vi "Exponential Test.vi"() -> ()   [LabVIEW 2014]
uses:
  <vilib>/Math Plots/3D Math Plots/3D Scatter/3D Scatter XCtrl/3D Scatter.xctl
  <vilib>/Math Plots/3D Math Plots/3D Scatter/3D Scatter Datatype/Public/Plot Helper (Vector).vi
  <vilib>/Analysis/1siggen.llb/Ramp Pattern by Delta.vi
  Math Utilities.lvlib
  <vilib>/Analysis/NI_AALBase.lvlib
  <vilib>/measure/NI_MABase.lvlib
  <vilib>/Math Plots/3D Math Plots/3D Scatter/3D Scatter Datatype/3D Scatter Datatype.lvclass
panel:
  in  "meth":enum8{"DFT-1", "DFT-5", "LRS"}(ring)=enum."LRS" caption="Exponential Fit Method"
  out "etau'":cluster{dbl[], dbl[]}[](graph)=[{[0.0, 0.05, 0.1, 0.15, 0.2, 0.25, 0.3, 0.35, 0.4, 0.45, 0.5, 0.55, 0.6, 0.65, 0.7, 0.75, 0.8, 0.85, 0.9, 0.95, 1.0, 1.05, 1.1, 1.15, 1.2, 1.25, 1.3, 1.35, 1.4, 1.45, 1.5, 1.55, 1.6, 1.65, 1.7, 1.75, 1.8, 1.85, 1.9, 1.95, 2.0, 2.05, 2.1, 2.15, 2.2, 2.25, 2.3, 2.35, 2.4, 2.45, 2.5, 2.55, 2.6, 2.65, 2.7, 2.75, 2.8, 2.85, 2.9, 2.95, 3.0, 3.05, 3.1, 3.15, 3.2, 3.25, 3.3, 3.35, 3.4, 3.45, 3.5, 3.55, 3.6, 3.65, 3.7, 3.75, 3.8, 3.85, 3.9, 3.95, 4.0, 4.05, 4.1, 4.15, 4.2, 4.25, 4.3, 4.35, 4.4, 4.45, 4.5, 4.55, 4.6, 4.65, 4.7, 4.75, 4.8, 4.85, 4.9, 4.95], [0.960541444934628, 1.0300287046137588, 0.8896412059372913, 0.8809320306793802, 0.7883247330312061, 0.8176833763391205, 0.6447128922258879, 0.6273332809368509, 0.6605682518837364, 0.6670014264280115, 0.583805564940926, 0.675732358744051, 0.4639846933111526, 0.6202542521121932, 0.5597277145279371, 0.5135564243561868, 0.5062733727780937, 0.3613578160271843, 0.4475233678516537, 0.3793968608808492, 0.43724877411342006, 0.3597384315625127, 0.2373620816547545, 0.22453592933762084, 0.29842459974751334, 0.3050071640074105, 0.2359236866011837, 0.24302284161365773, 0.23920428907537397, 0.2700720254736181, 0.1918881215092269, 0.2316375620963971, 0.2698374059004593, 0.10938565371609907, 0.18228368619733432, 0.1995904055680095, 0.10262683454287629, 0.12951323626014882, 0.1883316121198414, 0.051005880662942066, 0.1882658145929273, 0.2253474344702741, 0.1072676376138868, 0.05420331503554107, 0.07073686122149538, 0.19072834912888081, 0.06489404614590896, 0.02340665923857653, 0.080727031502262, 0.053160478621205834, 0.1150566849039812, 0.08647339206694683, 0.17225004999139676, 0.14385515421965545, 0.09476811084635094, 0.08535850566392958, 0.042453337460426295, -0.005111835078437502, 0.1266720101202937, 0.08798857698089546, 0.06448330591172151, 0.012535109492323698, -0.02180050629331399, 0.13921091410606592, -0.00448119475112807, 0.025953771409014427, 0.09196924940378937, 0.1251848736523793, 0.09872337746996236, -0.02796928416987523, -0.0439093646999277, 0.07577564143222511, -0.03469012345164275, 0.1000290582787502, 0.07570130581455305, 0.10981843839037647, 0.030883562880611268, 0.05482327411195698, -0.016277970417741722, 0.0739773731669493, 0.11823230258380474, 0.022378034520468177, 0.015118202748243353, 0.06436576688809863, 0.034369714129696256, -0.07590989562072355, 0.11223730777048424, -0.05352288298618646, 0.059251144916092124, -0.054463595365239675, 0.10903521158421503, 0.07349724843361212, -0.04763649889666532, 0.05840026342982382, -0.06312941047179772, -0.04841695002411584, 0.0871009289199655, -0.08241366972549377, 0.06657825659960447, 0.01870496404000565]}, {[0.0, 0.1, 0.2, 0.3, 0.4, 0.5, 0.6, 0.7, 0.8, 0.9, 1.0, 1.1, 1.2, 1.3, 1.4, 1.5, 1.6, 1.7, 1.8, 1.9, 2.0, 2.1, 2.2, 2.3, 2.4, 2.5, 2.6, 2.7, 2.8, 2.9, 3.0, 3.1, 3.2, 3.3, 3.4, 3.5, 3.6, 3.7, 3.8, 3.9, 4.0, 4.1, 4.2, 4.3, 4.4, 4.5, 4.6, 4.7, 4.8, 4.9], [1.0489118049155677, 0.9828657414468108, 0.7287092685494896, 0.7402604459878791, 0.5870346294794287, 0.586721816909444, 0.45440624030548527, 0.5237279303930864, 0.3972561140761981, 0.33254829917367884, 0.34818621735970484, 0.3989198005547301, 0.34947614865970883, 0.20883760536624074, 0.20965525245589398, 0.26857776347019313, 0.23122560558625996, 0.23874984457269088, 0.15561255360224382, 0.1418318343504817, 0.11626272362059906, 0.16392580193843515, 0.033834333279495796, 0.0778706880250746, -0.007929789367372514, 0.005419938340864641, 0.04836411782582296, 0.12887685022889384, 0.15987281329989583, 0.002826123372845442, 0.044361005460079386, 0.01107762227846102, 0.027130325332161268, -0.0329011607483985, -0.00976715691082395, -0.01851382955827155, -0.02912386416561294, 0.05216385233514075, -0.01890067181650635, -0.06324219670124576, -0.06851294508129749, -0.002777132357630538, -0.014512361417010615, 0.08683899542703284, 0.08258002031887463, -0.024344103284262092, 0.0437718075673618, -0.06155030056137617, 0.06644365751447188, 0.05045892575985402]}, {[0.0, 0.2, 0.4, 0.6, 0.8, 1.0, 1.2, 1.4, 1.6, 1.8, 2.0, 2.2, 2.4, 2.6, 2.8, 3.0, 3.2, 3.4, 3.6, 3.8, 4.0, 4.2, 4.4, 4.6, 4.8], [1.0166445888668472, 0.8965127205564365, 0.6746646020918559, 0.5979355379266843, 0.4854152133224972, 0.3872720439703156, 0.3657660253817956, 0.30351089738058307, 0.2198216708301479, 0.20705366479755255, 0.06903085210606028, 0.16530276730729707, 0.15939586940300982, 0.083518667159258, 0.0640925481270926, 0.06369433525293566, 0.04352509905837727, 0.036281546977637566, 0.043303657543107665, 0.08611682194308087, 0.029590496545093097, -0.01733169050921223, -0.024397551503856203, -0.05234666017391198, -0.03711380387257694]}, {[0.0, 0.5, 1.0, 1.5, 2.0, 2.5, 3.0, 3.5, 4.0, 4.5], [1.0623034361710997, 0.5317673867138099, 0.42771698929286195, 0.17661929472640508, 0.05033997654512429, 0.03973823954012479, 0.09664850852882598, 0.07924682307796599, 0.11213514888422532, 0.10083456799625037]}, {[0.0, 1.0, 2.0, 3.0, 4.0], [1.097092230716005, 0.32607780199041114, 0.13609726715261378, 0.0013463089040823967, 0.0574822313090591]}]
  out "tau'":cluster{dbl[], dbl[]}[](graph)=[{[0.0, 0.05, 0.1, 0.15, 0.2, 0.25, 0.3, 0.35, 0.4, 0.45, 0.5, 0.55, 0.6, 0.65, 0.7, 0.75, 0.8, 0.85, 0.9, 0.95, 1.0, 1.05, 1.1, 1.15, 1.2, 1.25, 1.3, 1.35, 1.4, 1.45, 1.5, 1.55, 1.6, 1.65, 1.7, 1.75, 1.8, 1.85, 1.9, 1.95, 2.0, 2.05, 2.1, 2.15, 2.2, 2.25, 2.3, 2.35, 2.4, 2.45, 2.5, 2.55, 2.6, 2.65, 2.7, 2.75, 2.8, 2.85, 2.9, 2.95, 3.0, 3.05, 3.1, 3.15, 3.2, 3.25, 3.3, 3.35, 3.4, 3.45, 3.5, 3.55, 3.6, 3.65, 3.7, 3.75, 3.8, 3.85, 3.9, 3.95, 4.0, 4.05, 4.1, 4.15, 4.2, 4.25, 4.3, 4.35, 4.4, 4.45, 4.5, 4.55, 4.6, 4.65, 4.7, 4.75, 4.8, 4.85, 4.9, 4.95], [0.960541444934628, 1.0300287046137588, 0.8896412059372913, 0.8809320306793802, 0.7883247330312061, 0.8176833763391205, 0.6447128922258879, 0.6273332809368509, 0.6605682518837364, 0.6670014264280115, 0.583805564940926, 0.675732358744051, 0.4639846933111526, 0.6202542521121932, 0.5597277145279371, 0.5135564243561868, 0.5062733727780937, 0.3613578160271843, 0.4475233678516537, 0.3793968608808492, 0.43724877411342006, 0.3597384315625127, 0.2373620816547545, 0.22453592933762084, 0.29842459974751334, 0.3050071640074105, 0.2359236866011837, 0.24302284161365773, 0.23920428907537397, 0.2700720254736181, 0.1918881215092269, 0.2316375620963971, 0.2698374059004593, 0.10938565371609907, 0.18228368619733432, 0.1995904055680095, 0.10262683454287629, 0.12951323626014882, 0.1883316121198414, 0.051005880662942066, 0.1882658145929273, 0.2253474344702741, 0.1072676376138868, 0.05420331503554107, 0.07073686122149538, 0.19072834912888081, 0.06489404614590896, 0.02340665923857653, 0.080727031502262, 0.053160478621205834, 0.1150566849039812, 0.08647339206694683, 0.17225004999139676, 0.14385515421965545, 0.09476811084635094, 0.08535850566392958, 0.042453337460426295, -0.005111835078437502, 0.1266720101202937, 0.08798857698089546, 0.06448330591172151, 0.012535109492323698, -0.02180050629331399, 0.13921091410606592, -0.00448119475112807, 0.025953771409014427, 0.09196924940378937, 0.1251848736523793, 0.09872337746996236, -0.02796928416987523, -0.0439093646999277, 0.07577564143222511, -0.03469012345164275, 0.1000290582787502, 0.07570130581455305, 0.10981843839037647, 0.030883562880611268, 0.05482327411195698, -0.016277970417741722, 0.0739773731669493, 0.11823230258380474, 0.022378034520468177, 0.015118202748243353, 0.06436576688809863, 0.034369714129696256, -0.07590989562072355, 0.11223730777048424, -0.05352288298618646, 0.059251144916092124, -0.054463595365239675, 0.10903521158421503, 0.07349724843361212, -0.04763649889666532, 0.05840026342982382, -0.06312941047179772, -0.04841695002411584, 0.0871009289199655, -0.08241366972549377, 0.06657825659960447, 0.01870496404000565]}, {[0.0, 0.1, 0.2, 0.3, 0.4, 0.5, 0.6, 0.7, 0.8, 0.9, 1.0, 1.1, 1.2, 1.3, 1.4, 1.5, 1.6, 1.7, 1.8, 1.9, 2.0, 2.1, 2.2, 2.3, 2.4, 2.5, 2.6, 2.7, 2.8, 2.9, 3.0, 3.1, 3.2, 3.3, 3.4, 3.5, 3.6, 3.7, 3.8, 3.9, 4.0, 4.1, 4.2, 4.3, 4.4, 4.5, 4.6, 4.7, 4.8, 4.9], [1.0489118049155677, 0.9828657414468108, 0.7287092685494896, 0.7402604459878791, 0.5870346294794287, 0.586721816909444, 0.45440624030548527, 0.5237279303930864, 0.3972561140761981, 0.33254829917367884, 0.34818621735970484, 0.3989198005547301, 0.34947614865970883, 0.20883760536624074, 0.20965525245589398, 0.26857776347019313, 0.23122560558625996, 0.23874984457269088, 0.15561255360224382, 0.1418318343504817, 0.11626272362059906, 0.16392580193843515, 0.033834333279495796, 0.0778706880250746, -0.007929789367372514, 0.005419938340864641, 0.04836411782582296, 0.12887685022889384, 0.15987281329989583, 0.002826123372845442, 0.044361005460079386, 0.01107762227846102, 0.027130325332161268, -0.0329011607483985, -0.00976715691082395, -0.01851382955827155, -0.02912386416561294, 0.05216385233514075, -0.01890067181650635, -0.06324219670124576, -0.06851294508129749, -0.002777132357630538, -0.014512361417010615, 0.08683899542703284, 0.08258002031887463, -0.024344103284262092, 0.0437718075673618, -0.06155030056137617, 0.06644365751447188, 0.05045892575985402]}, {[0.0, 0.2, 0.4, 0.6, 0.8, 1.0, 1.2, 1.4, 1.6, 1.8, 2.0, 2.2, 2.4, 2.6, 2.8, 3.0, 3.2, 3.4, 3.6, 3.8, 4.0, 4.2, 4.4, 4.6, 4.8], [1.0166445888668472, 0.8965127205564365, 0.6746646020918559, 0.5979355379266843, 0.4854152133224972, 0.3872720439703156, 0.3657660253817956, 0.30351089738058307, 0.2198216708301479, 0.20705366479755255, 0.06903085210606028, 0.16530276730729707, 0.15939586940300982, 0.083518667159258, 0.0640925481270926, 0.06369433525293566, 0.04352509905837727, 0.036281546977637566, 0.043303657543107665, 0.08611682194308087, 0.029590496545093097, -0.01733169050921223, -0.024397551503856203, -0.05234666017391198, -0.03711380387257694]}, {[0.0, 0.5, 1.0, 1.5, 2.0, 2.5, 3.0, 3.5, 4.0, 4.5], [1.0623034361710997, 0.5317673867138099, 0.42771698929286195, 0.17661929472640508, 0.05033997654512429, 0.03973823954012479, 0.09664850852882598, 0.07924682307796599, 0.11213514888422532, 0.10083456799625037]}, {[0.0, 1.0, 2.0, 3.0, 4.0], [1.097092230716005, 0.32607780199041114, 0.13609726715261378, 0.0013463089040823967, 0.0574822313090591]}]
  out "3D Scatter":refnum<class "3D Plot Datatype.lvclass">[](xcontrol)
  out "CalcData":T1(array[cluster])
  in  "taus":dbl[](array[numeric])=[0.5, 1.0, 2.0, 5.0, 10.0, 20.0, 50.0, 100.0, 150.0] caption="taus (us)"
  in  "noise":dbl[](array[numeric])=[0.0, 0.01, 0.05, 0.1, 0.2, 0.3, 0.4, 0.5, 1.0] caption="Noise Levels"
  in  "Ntaus":dbl=5.0 caption="# Taus"
  in  "Nsamp":dbl=4000.0 caption="Number of Samples"
  out "Taus":T2(graph)=[{"Sampling Frequencies (MHz)"=[20.0, 10.0, 5.0, 2.0, 1.0], [0.9656086307823587, 0.9866685202887719, 1.1569644501410312, 0.7662051282812012, 0.8285928880796682]}, {"Sampling Frequencies (MHz)"=[20.0, 10.0, 5.0, 2.0, 1.0], [0.026104009183676023, 0.034896410998791996, 0.03328061139393245, 0.07782595805221088, 0.07635392209771198]}, {"Sampling Frequencies (MHz)"=[20.0, 10.0, 5.0, 2.0, 1.0], [0.9408079235146063, 0.9408079235146063, 0.9408079235146063, 0.9408079235146063, 0.9408079235146063]}]
  out "Exponential":cluster{dbl[], dbl[]}[](graph)=[{[0.0, 0.05, 0.1, 0.15, 0.2, 0.25, 0.3, 0.35, 0.4, 0.45, 0.5, 0.55, 0.6, 0.65, 0.7, 0.75, 0.8, 0.85, 0.9, 0.95, 1.0, 1.05, 1.1, 1.15, 1.2, 1.25, 1.3, 1.35, 1.4, 1.45, 1.5, 1.55, 1.6, 1.65, 1.7, 1.75, 1.8, 1.85, 1.9, 1.95, 2.0, 2.05, 2.1, 2.15, 2.2, 2.25, 2.3, 2.35, 2.4, 2.45, 2.5, 2.55, 2.6, 2.65, 2.7, 2.75, 2.8, 2.85, 2.9, 2.95, 3.0, 3.05, 3.1, 3.15, 3.2, 3.25, 3.3, 3.35, 3.4, 3.45, 3.5, 3.55, 3.6, 3.65, 3.7, 3.75, 3.8, 3.85, 3.9, 3.95, 4.0, 4.05, 4.1, 4.15, 4.2, 4.25, 4.3, 4.35, 4.4, 4.45, 4.5, 4.55, 4.6, 4.65, 4.7, 4.75, 4.8, 4.85, 4.9, 4.95], [0.960541444934628, 1.0300287046137588, 0.8896412059372913, 0.8809320306793802, 0.7883247330312061, 0.8176833763391205, 0.6447128922258879, 0.6273332809368509, 0.6605682518837364, 0.6670014264280115, 0.583805564940926, 0.675732358744051, 0.4639846933111526, 0.6202542521121932, 0.5597277145279371, 0.5135564243561868, 0.5062733727780937, 0.3613578160271843, 0.4475233678516537, 0.3793968608808492, 0.43724877411342006, 0.3597384315625127, 0.2373620816547545, 0.22453592933762084, 0.29842459974751334, 0.3050071640074105, 0.2359236866011837, 0.24302284161365773, 0.23920428907537397, 0.2700720254736181, 0.1918881215092269, 0.2316375620963971, 0.2698374059004593, 0.10938565371609907, 0.18228368619733432, 0.1995904055680095, 0.10262683454287629, 0.12951323626014882, 0.1883316121198414, 0.051005880662942066, 0.1882658145929273, 0.2253474344702741, 0.1072676376138868, 0.05420331503554107, 0.07073686122149538, 0.19072834912888081, 0.06489404614590896, 0.02340665923857653, 0.080727031502262, 0.053160478621205834, 0.1150566849039812, 0.08647339206694683, 0.17225004999139676, 0.14385515421965545, 0.09476811084635094, 0.08535850566392958, 0.042453337460426295, -0.005111835078437502, 0.1266720101202937, 0.08798857698089546, 0.06448330591172151, 0.012535109492323698, -0.02180050629331399, 0.13921091410606592, -0.00448119475112807, 0.025953771409014427, 0.09196924940378937, 0.1251848736523793, 0.09872337746996236, -0.02796928416987523, -0.0439093646999277, 0.07577564143222511, -0.03469012345164275, 0.1000290582787502, 0.07570130581455305, 0.10981843839037647, 0.030883562880611268, 0.05482327411195698, -0.016277970417741722, 0.0739773731669493, 0.11823230258380474, 0.022378034520468177, 0.015118202748243353, 0.06436576688809863, 0.034369714129696256, -0.07590989562072355, 0.11223730777048424, -0.05352288298618646, 0.059251144916092124, -0.054463595365239675, 0.10903521158421503, 0.07349724843361212, -0.04763649889666532, 0.05840026342982382, -0.06312941047179772, -0.04841695002411584, 0.0871009289199655, -0.08241366972549377, 0.06657825659960447, 0.01870496404000565]}, {[0.0, 0.1, 0.2, 0.3, 0.4, 0.5, 0.6, 0.7, 0.8, 0.9, 1.0, 1.1, 1.2, 1.3, 1.4, 1.5, 1.6, 1.7, 1.8, 1.9, 2.0, 2.1, 2.2, 2.3, 2.4, 2.5, 2.6, 2.7, 2.8, 2.9, 3.0, 3.1, 3.2, 3.3, 3.4, 3.5, 3.6, 3.7, 3.8, 3.9, 4.0, 4.1, 4.2, 4.3, 4.4, 4.5, 4.6, 4.7, 4.8, 4.9], [1.0489118049155677, 0.9828657414468108, 0.7287092685494896, 0.7402604459878791, 0.5870346294794287, 0.586721816909444, 0.45440624030548527, 0.5237279303930864, 0.3972561140761981, 0.33254829917367884, 0.34818621735970484, 0.3989198005547301, 0.34947614865970883, 0.20883760536624074, 0.20965525245589398, 0.26857776347019313, 0.23122560558625996, 0.23874984457269088, 0.15561255360224382, 0.1418318343504817, 0.11626272362059906, 0.16392580193843515, 0.033834333279495796, 0.0778706880250746, -0.007929789367372514, 0.005419938340864641, 0.04836411782582296, 0.12887685022889384, 0.15987281329989583, 0.002826123372845442, 0.044361005460079386, 0.01107762227846102, 0.027130325332161268, -0.0329011607483985, -0.00976715691082395, -0.01851382955827155, -0.02912386416561294, 0.05216385233514075, -0.01890067181650635, -0.06324219670124576, -0.06851294508129749, -0.002777132357630538, -0.014512361417010615, 0.08683899542703284, 0.08258002031887463, -0.024344103284262092, 0.0437718075673618, -0.06155030056137617, 0.06644365751447188, 0.05045892575985402]}, {[0.0, 0.2, 0.4, 0.6, 0.8, 1.0, 1.2, 1.4, 1.6, 1.8, 2.0, 2.2, 2.4, 2.6, 2.8, 3.0, 3.2, 3.4, 3.6, 3.8, 4.0, 4.2, 4.4, 4.6, 4.8], [1.0166445888668472, 0.8965127205564365, 0.6746646020918559, 0.5979355379266843, 0.4854152133224972, 0.3872720439703156, 0.3657660253817956, 0.30351089738058307, 0.2198216708301479, 0.20705366479755255, 0.06903085210606028, 0.16530276730729707, 0.15939586940300982, 0.083518667159258, 0.0640925481270926, 0.06369433525293566, 0.04352509905837727, 0.036281546977637566, 0.043303657543107665, 0.08611682194308087, 0.029590496545093097, -0.01733169050921223, -0.024397551503856203, -0.05234666017391198, -0.03711380387257694]}, {[0.0, 0.5, 1.0, 1.5, 2.0, 2.5, 3.0, 3.5, 4.0, 4.5], [1.0623034361710997, 0.5317673867138099, 0.42771698929286195, 0.17661929472640508, 0.05033997654512429, 0.03973823954012479, 0.09664850852882598, 0.07924682307796599, 0.11213514888422532, 0.10083456799625037]}, {[0.0, 1.0, 2.0, 3.0, 4.0], [1.097092230716005, 0.32607780199041114, 0.13609726715261378, 0.0013463089040823967, 0.0574822313090591]}]
  in  "B":dbl
  in  "A":dbl=1.0
  in  "fsamp":dbl[](array[numeric])=[20.0, 15.0, 10.0, 8.0, 6.0, 5.0, 2.5, 1.0] caption="Sampling Frequencies (MHz)"
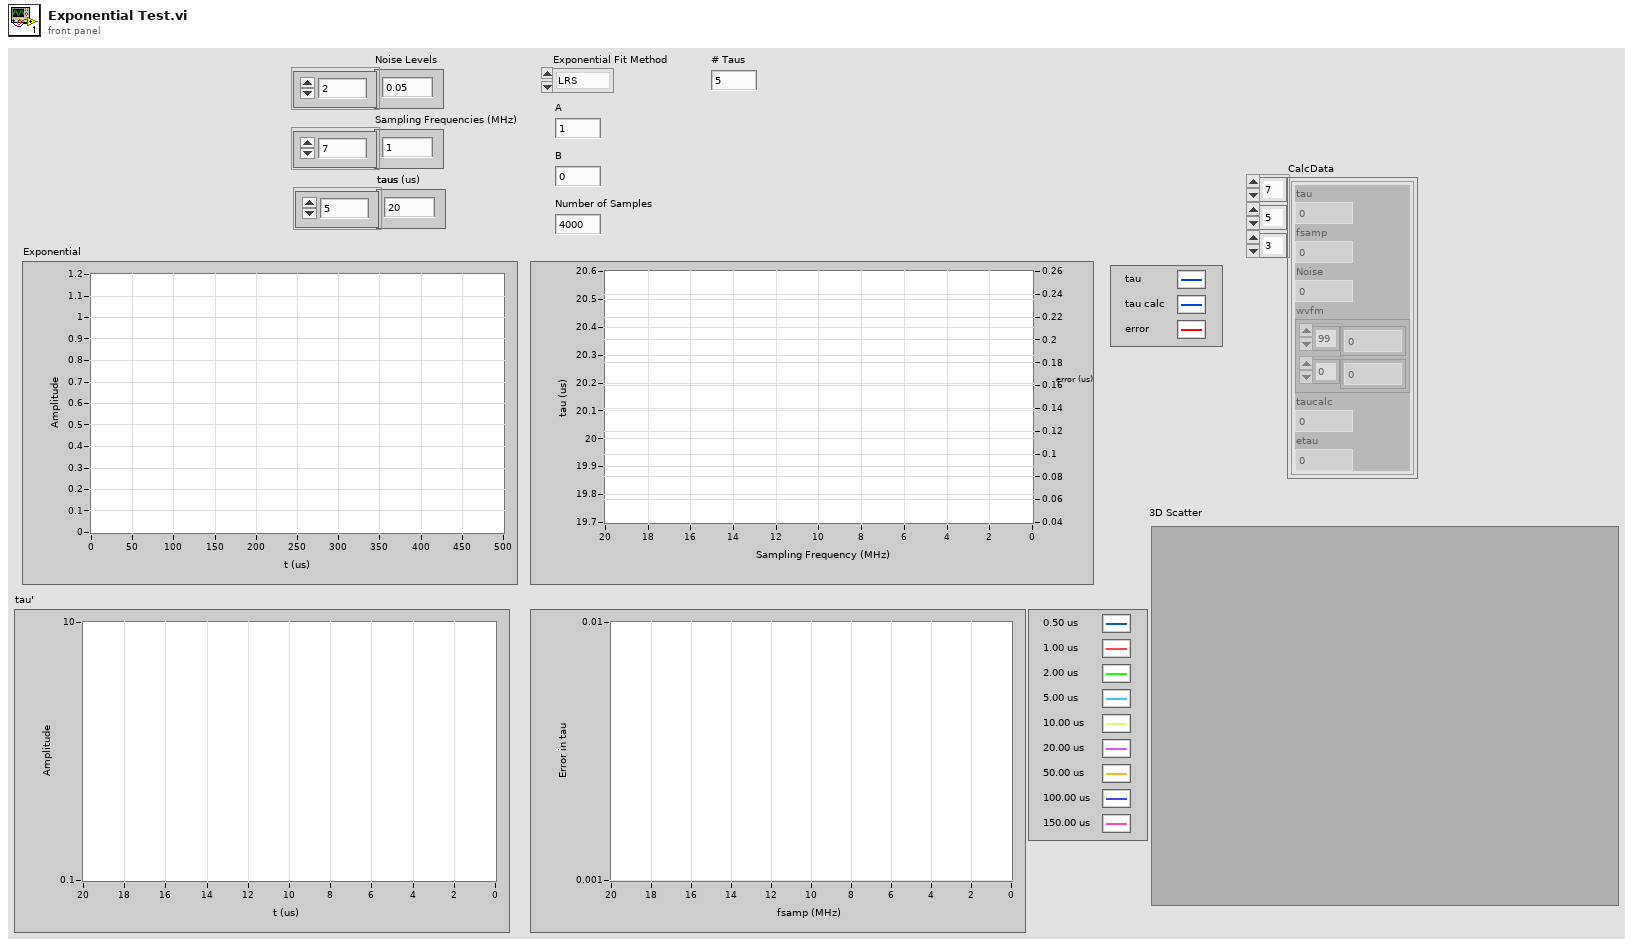
[diagram p1: front panel]
types:
  T1 = cluster{"tau":dbl, "fsamp":dbl, "Noise":dbl, "wvfm":cluster{dbl[], dbl[]}, "taucalc":dbl, "etau":dbl}[][][]
  T2 = cluster{"Sampling Frequencies (MHz)":dbl[], dbl[]}[]
  T3 = cluster{dbl, dbl, "Numeric":dbl, cluster{dbl[], dbl[]}, "tau":dbl, "e_tau":dbl}[][][]
  T4 = cluster{"tau":dbl, "fsamp":dbl, "Noise":dbl, "wvfm":cluster{dbl[], dbl[]}, "taucalc":dbl, "etau":dbl}
  T5 = cluster{"tau":dbl, "fsamp":dbl, "Noise":dbl, "wvfm":cluster{dbl[], dbl[]}, "taucalc":dbl, "etau":dbl}[][]
  T6 = cluster{"tau":dbl, "fsamp":dbl, "Noise":dbl, "wvfm":cluster{dbl[], dbl[]}, "taucalc":dbl, "etau":dbl}[]
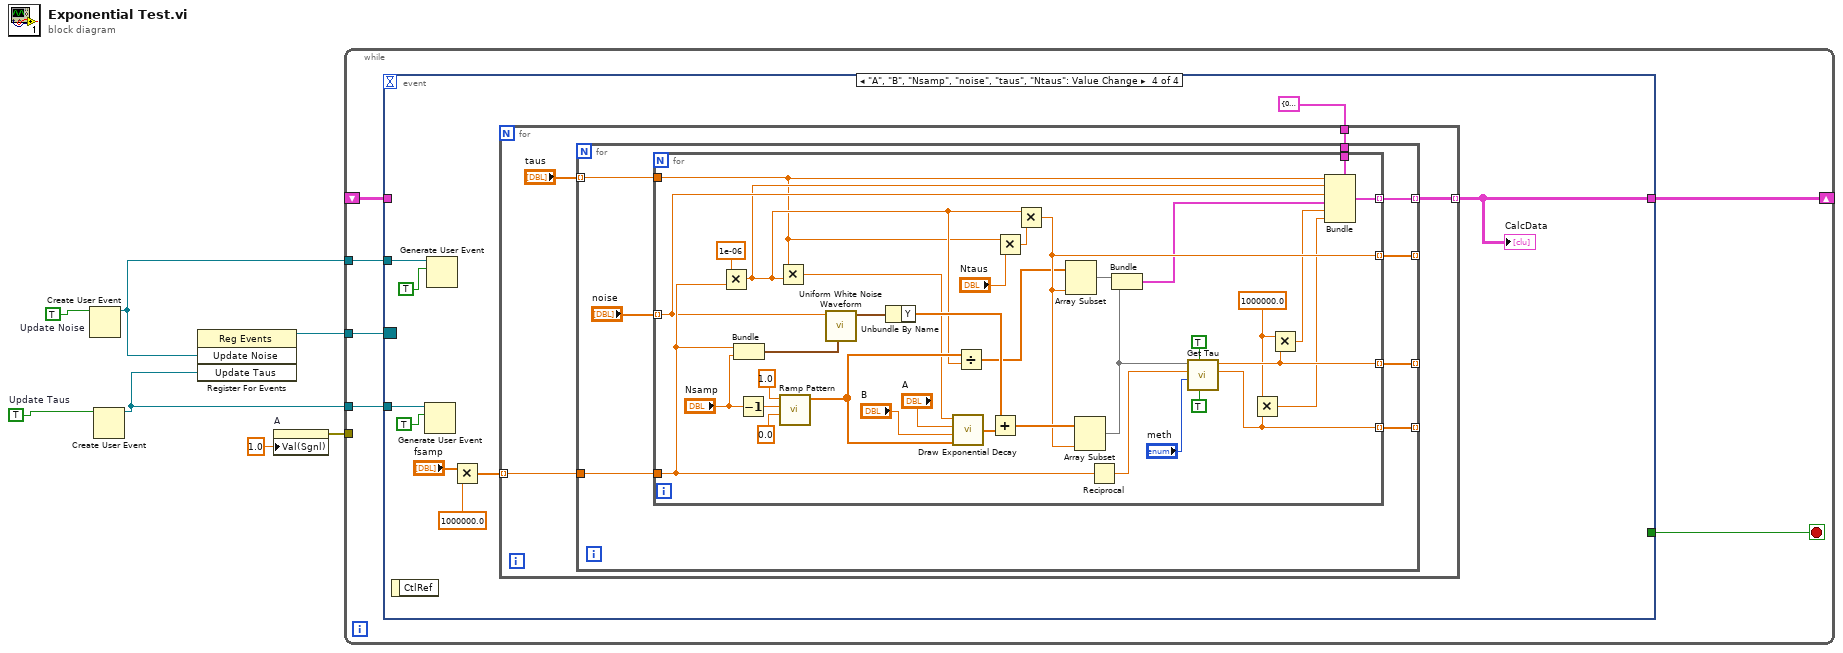
[diagram p0: block diagram]
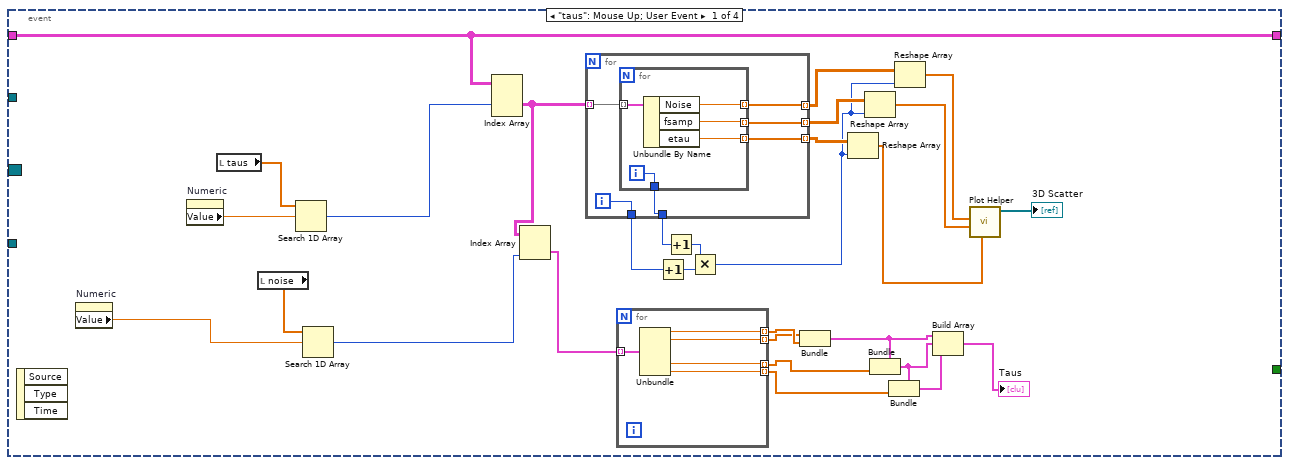
[diagram p2: hidden frame]
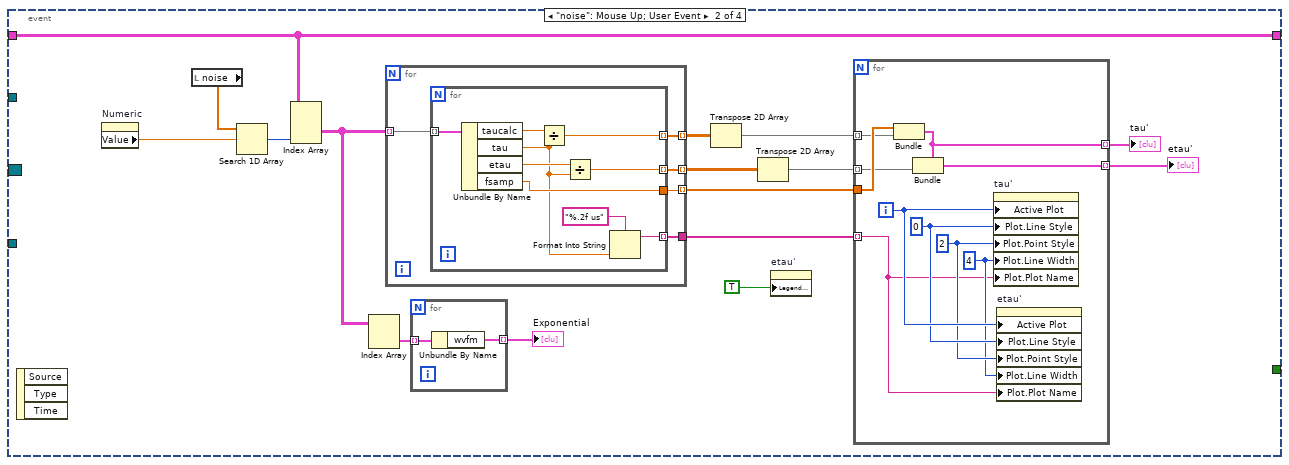
[diagram p3: hidden frame]
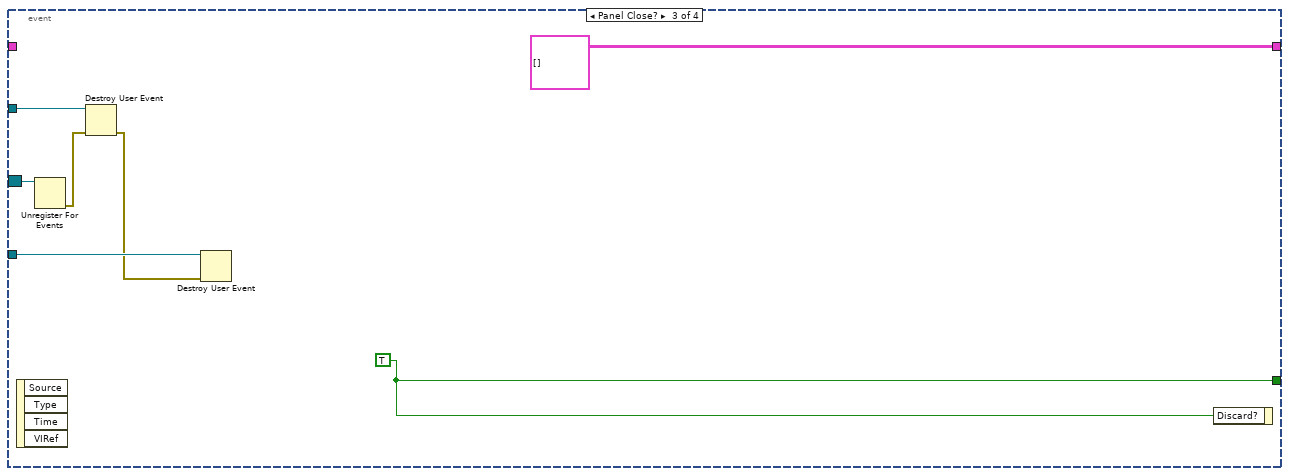
[diagram p4: hidden frame]
diagram:
  w2 = TRUE  # Update Taus
  w5 = TRUE  # Update Noise
  n1 = Create User Event(user event datatype=w5) -> (user event=w3:refnum<user-event>)  [unwired: 1 in, 1 out]
  n2 = Create User Event(user event datatype=w2) -> (user event=w1:refnum<user-event>)  [unwired: 1 in, 1 out]
  n3 = register-events(w3, w1) -> (reference out=w4:refnum<event-registration>)  [unwired: 2 in, 1 out]
  n4 = property on="A" class="DigNum (strict)"("Val(Sgnl)"=1.0 ("Value (Signaling)")) -> (error out=w6:errorcluster)  [unwired: 2 in, 1 out]
  n5 = while {
    shift-right: [w12] -> _
    shift-left: _ -> [w11]
    tunnel: w6 -> [_]
    tunnel: w4 -> [w10]
    tunnel: w3 -> [w9]
    tunnel: w1 -> [w8]
    stop <- w13 stop-if-true
    n6 = event shown="[3] \"A\", \"B\", \"Nsamp\", \"noise\", \"taus\", \"Ntaus\": Value Change" {
      selector: w10 -> [_ _ w103 _]
      dyn-events: _ -> [_ _ _ _]
      timeout: _ -> [_ _ _ _]
      tunnel: [_ _ w107 _] -> w13
      tunnel: [w42 w74 T3 [] w111] -> w12
      tunnel: w11 -> [w42 w74 _ _]
      tunnel: w9 -> [_ _ w104 w113]
      tunnel: w8 -> [_ _ w105 w110]
      event "taus": Mouse Up; User Event {
        n7 = event-data() -> ()  [unwired: 1 in, 3 out]
        n8 = property on="Numeric" class="DigNum (strict)"() -> ("Value"=w26:dbl)  [unwired: 2 in, 2 out]
        n9 = property on="Numeric" class="DigNum (strict)"() -> ("Value"=w28:dbl)  [unwired: 2 in, 2 out]
        n10 = local read "taus"() -> (w29:dbl[])
        n11 = local read "noise"() -> (w25:dbl[])
        n12 = Search 1D Array(1D array=w29, element=w28) -> (index of element=w27:i32)  [unwired: 1 in]
        n13 = Search 1D Array(1D array=w25, element=w26) -> (index of element=w23:i32)  [unwired: 1 in]
        n14 = Index Array(array=w42, index (dim 1)=w27) -> (element=w24:T5)  [unwired: 2 in]
        n15 = Index Array(array=w24, index (col)=w23) -> (element=w22:T6)  [unwired: 1 in]
        n16 = for {
          tunnel: w24 -> [w53] mode=indexing
          tunnel: [w52] -> w36 mode=indexing
          tunnel: [w51] -> w34 mode=indexing
          tunnel: [w50] -> w41 mode=indexing
          tunnel: [w49] -> w39
          tunnel: [w48] -> w40
          i -> [w48]
          n17 = for {
            tunnel: w53 -> [w58] mode=indexing
            tunnel: [w57] -> w51 mode=indexing
            tunnel: [w56] -> w52 mode=indexing
            tunnel: [w55] -> w50 mode=indexing
            tunnel: [w54] -> w49
            i -> [w54]
            n18 = Unbundle By Name(w58) -> ("Noise"=w57:dbl, "fsamp"=w56:dbl, "etau"=w55:dbl)
          }
        }
        n19 = for {
          tunnel: w22 -> [w47] mode=indexing
          tunnel: [w46] -> w21 mode=indexing
          tunnel: [w45] -> w20 mode=indexing
          tunnel: [w44] -> w19 mode=indexing
          tunnel: [w43] -> w18 mode=indexing
          n20 = Unbundle(w47) -> ("tau"=w46:dbl, "fsamp"=w45:dbl, "taucalc"=w44:dbl, "etau"=w43:dbl)  [unwired: 2 out]
        }
        n21 = Increment(x=w40) -> (x+1=w37:i32)
        n22 = Increment(x=w39) -> (x+1=w38:i32)
        n23 = Multiply(x=w38, y=w37) -> (x*y=w35:i32)
        n24 = Bundle(w20, w21) -> (w17:cluster{dbl[], dbl[]})  [unwired: 1 in]
        n25 = Reshape Array(w41, w35) -> (w32:dbl[])
        n26 = Reshape Array(w36, w35) -> (w30:dbl[])
        n27 = Bundle(cluster=w17, w19) -> (w16:cluster{dbl[], dbl[]})  [unwired: 1 in]
        n28 = Bundle(cluster=w16, w18) -> (w15:cluster{dbl[], dbl[]})  [unwired: 1 in]
        n29 = Reshape Array(w34, w35) -> (w31:dbl[])
        n30 = Build Array(w17, w16, w15) -> (→"Taus":cluster{dbl[], dbl[]}[])
        n31 = call-poly <vilib>:"Plot Helper.vi"("z vector"=w32, "y vector"=w30, "x vector"=w31) -> ("3D Plot lvclass Array out"=→"3D Scatter":refnum<class "3D Plot Datatype.lvclass">[])  [unwired: 3 in, 5 out]
      }
      event "noise": Mouse Up; User Event {
        n32 = event-data() -> ()  [unwired: 1 in, 3 out]
        n33 = property on="Numeric" class="DigNum (strict)"() -> ("Value"=w61:dbl)  [unwired: 2 in, 2 out]
        n34 = local read "noise"() -> (w60:dbl[])
        n35 = Search 1D Array(1D array=w60, element=w61) -> (index of element=w59:i32)  [unwired: 1 in]
        n36 = Index Array(array=w74, index (dim 2)=w59) -> (element=w64:T5)  [unwired: 2 in]
        n37 = Index Array(array=w64) -> (element=w63:T6)  [unwired: 2 in]
        n38 = for {
          tunnel: w64 -> [w91] mode=indexing
          tunnel: [w90] -> w73 mode=indexing
          tunnel: [w89] -> w72 mode=indexing
          tunnel: [w88] -> w69 mode=indexing
          tunnel: [w87] -> w65
          n39 = for {
            tunnel: w91 -> [w100] mode=indexing
            tunnel: [w96] -> w90 mode=indexing
            tunnel: [w98] -> w89 mode=indexing
            tunnel: [w97] -> w88
            tunnel: [w94] -> w87 mode=indexing
            n40 = Unbundle By Name(w100) -> ("taucalc"=w93:dbl, "tau"=w92:dbl, "etau"=w99:dbl, "fsamp"=w97:dbl)
            n41 = Divide(x=w93, y=w92) -> (x/y=w96:dbl)
            n42 = Divide(x=w99, y=w92) -> (x/y=w98:dbl)
            n43 = Format Into String(format string="%.2f us", w92) -> (resulting string=w94:string)  [unwired: 2 in, 1 out]
          }
        }
        n44 = for {
          tunnel: w63 -> [w76] mode=indexing
          tunnel: [w75] -> w62 mode=indexing
          n45 = Unbundle By Name(w76) -> ("wvfm"=w75:cluster{dbl[], dbl[]})
        }
        "Exponential" <- w62
        n46 = Transpose 2D Array(2D array=w73) -> (transposed array=w71:dbl[][])
        n47 = Transpose 2D Array(2D array=w72) -> (transposed array=w70:dbl[][])
        n48 = property on="etau'" class="XYGraph (strict)"("Legend Visible"=TRUE ("Legend:Visible")) -> ()  [unwired: 2 in, 2 out]
        n49 = for {
          tunnel: w71 -> [w85] mode=indexing
          tunnel: w70 -> [w84] mode=indexing
          tunnel: w69 -> [w86]
          tunnel: [w83] -> w67 mode=indexing
          tunnel: [w82] -> w68 mode=indexing
          tunnel: w65 -> [w77] mode=indexing
          i -> [w81]
          w78 = u8 4 ("Plot.Line Width")
          w79 = u8 2 ("Plot.Point Style")
          w80 = u8 0 ("Plot.Line Style")
          n50 = Bundle(w86, w85) -> (w82:cluster{dbl[], dbl[]})  [unwired: 1 in]
          n51 = Bundle(cluster=w82, w84) -> (w83:cluster{dbl[], dbl[]})  [unwired: 1 in]
          n52 = property on="tau'" class="XYGraph (strict)"("Active Plot"=w81, "Plot.Line Style"=w80, "Plot.Point Style"=w79, "Plot.Line Width"=w78, "Plot.Plot Name"=w77) -> ()  [unwired: 2 in, 2 out]
          n53 = property on="etau'" class="XYGraph (strict)"("Active Plot"=w81, "Plot.Line Style"=w80, "Plot.Point Style"=w79, "Plot.Line Width"=w78, "Plot.Plot Name"=w77) -> ()  [unwired: 2 in, 2 out]
        }
        "tau'" <- w68
        "etau'" <- w67
      }
      event Panel Close? {
        w107 = TRUE ("Discard?")
        n54 = event-data() -> ()  [unwired: 1 in, 4 out]
        n55 = Unregister For Events(event registration refnum=w103) -> (error out=w102:errorcluster)  [unwired: 1 in]
        n56 = Destroy User Event(user event=w104, error in=w102) -> (error out=w101:errorcluster)
        n57 = Destroy User Event(user event=w105, error in=w101) -> ()  [unwired: 1 out]
        n58 = event-data("Discard?"=w107) -> ()  [unwired: 1 in, 1 out]
      }
      event "A", "B", "Nsamp", "noise", "taus", "Ntaus": Value Change {
        n59 = event-data() -> ()  [unwired: 1 in, 1 out]
        n60 = Generate User Event(user event=w110, event data cluster=TRUE ("event data")) -> ()  [unwired: 2 in, 2 out]
        n61 = Generate User Event(user event=w113, event data cluster=TRUE ("event data")) -> ()  [unwired: 2 in, 2 out]
        n62 = Multiply(x="fsamp", y=1000000.0 ("Numeric")) -> (x*y=w116:dbl[])
        n63 = for {
          tunnel: w116 -> [w120] mode=indexing
          tunnel: [w118] -> w111 mode=indexing
          tunnel: T4 {"tau"=0.0, "fsamp"=0.0, "Noise"=0.0, "wvfm"={[], []}, "taucalc"=0.0, "etau"=0.0} ("cluster") -> [w117]
          n64 = for {
            tunnel: "taus" -> [w128] mode=indexing
            tunnel: w120 -> [w127]
            tunnel: [w126] -> _ mode=indexing
            tunnel: [w125] -> _ mode=indexing
            tunnel: [w124] -> _ mode=indexing
            tunnel: [w122] -> w118 mode=indexing
            tunnel: w117 -> [w121]
            n65 = for {
              tunnel: "noise" -> [w143] mode=indexing
              tunnel: [w139] -> w126 mode=indexing
              tunnel: [w137] -> w125 mode=indexing
              tunnel: w128 -> [w133]
              tunnel: [w149] -> w124 mode=indexing
              tunnel: w127 -> [w145]
              tunnel: [w140] -> w122 mode=indexing
              tunnel: w121 -> [w134]
              w136 = 1000000.0 ("Numeric")
              n66 = Multiply(x=1e-06, y=w145) -> (x*y=w142:dbl)
              n67 = Bundle("Numeric"=w145, "Nsamp"="Nsamp") -> (w161:cluster{"Numeric":dbl, "Nsamp":dbl})  [unwired: 1 in]
              n68 = Decrement(x="Nsamp") -> (x-1=w158:dbl)
              n69 = Multiply(x=w133, y=w142) -> (x*y=w144:dbl)
              n70 = call-poly <vilib>:"Ramp Pattern.vi"("start"=0.0, "end"=w158, "delta"=1.0) -> ("Ramp Pattern"=w156:dbl[])  [unwired: 6 in, 2 out]
              n71 = call <vilib>:"Uniform White Noise Waveform.vi"("sampling info"=w161, "amplitude"=w143) -> ("signal out"=w162:waveform(dbl))  [unwired: 8 in, 1 out]
              n72 = Unbundle By Name(w162) -> ("Y"=w159:dbl[])
              n73 = call "Draw Exponential Decay.vi"("time"=w156, "B"="B", "A"="A", "tau"=w144) -> ("ExponentialOut"=w160:dbl[])
              n74 = Divide(x=w156, y=w142) -> (x/y=w148:dbl[])
              n75 = Add(x=w159, y=w160) -> (x+y=w150:dbl[])
              n76 = Multiply(x=w133, y="Ntaus") -> (x*y=w152:dbl)
              n77 = Multiply(x=w142, y=w152) -> (x*y=w149:dbl)
              n78 = Array Subset(array=w148, length=w149) -> (w147:dbl[])  [unwired: 1 in]
              n79 = Array Subset(array=w150, length=w149) -> (w146:dbl[])  [unwired: 1 in]
              n80 = Reciprocal(x=w145) -> (1/x=w155:dbl)
              n81 = Bundle(w147, w146) -> (w141:cluster{dbl[], dbl[]})  [unwired: 1 in]
              n82 = call "Get Tau.vi"("ErrorCallOn"=TRUE, "init"=TRUE, "CalType"="meth", "Dt"=w155, "X"=w146) -> ("e_tau"=w137:dbl, "tau"=w139:dbl)  [unwired: 3 in, 2 out]
              n83 = Multiply(x=w136, y=w137) -> (x*y=w135:dbl)
              n84 = Multiply(x=w136, y=w139) -> (x*y=w138:dbl)
              n85 = Bundle(cluster=w134, "tau"=w133, "fsamp"=w142, "Noise"=w143, "wvfm"=w141, "taucalc"=w138, "etau"=w135) -> (w140:T4)
            }
          }
        }
        "CalcData" <- w111
      }
    }
  }
